vi "SVI_SerialSendAndReceive.vi"(6 "End Char":string="\n", 7 "Wait time (ms)":u32=1000, 8 "error in (no error)":errorcluster, 9 "Tries":i32=50, 10 "Command":string, 11 "VISA Refnum in":refnum<visa-resource-name>) -> (0 "error out":errorcluster, 2 "read buffer":string, 3 "VISA resource name out":refnum<visa-resource-name>)   [LabVIEW 2014]
panel:
  out "Numeric Control":i32
  out "Array":u32[](array[numeric])
  out "Tries":i32
  out "x-y":u32
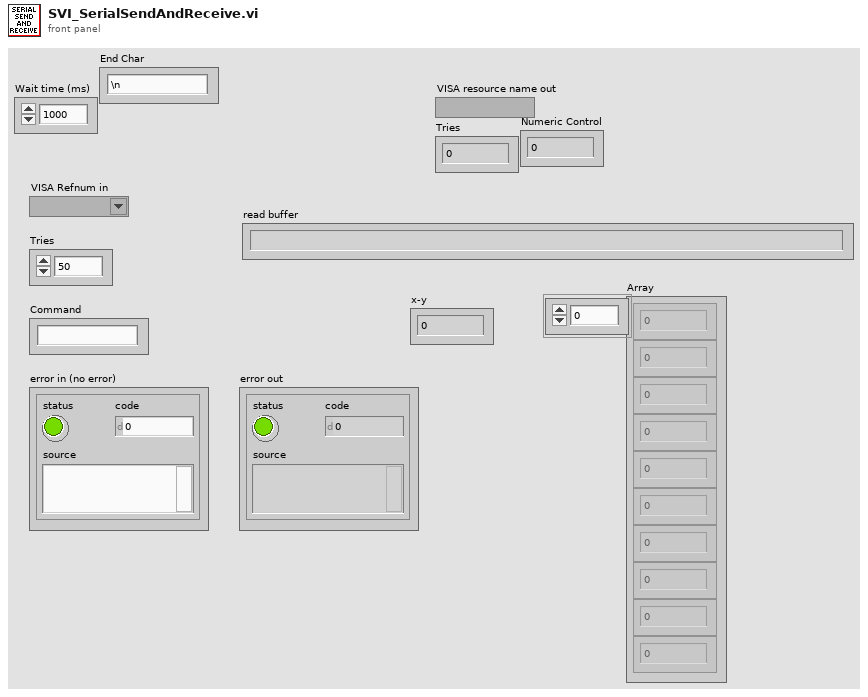
[diagram p1: front panel]
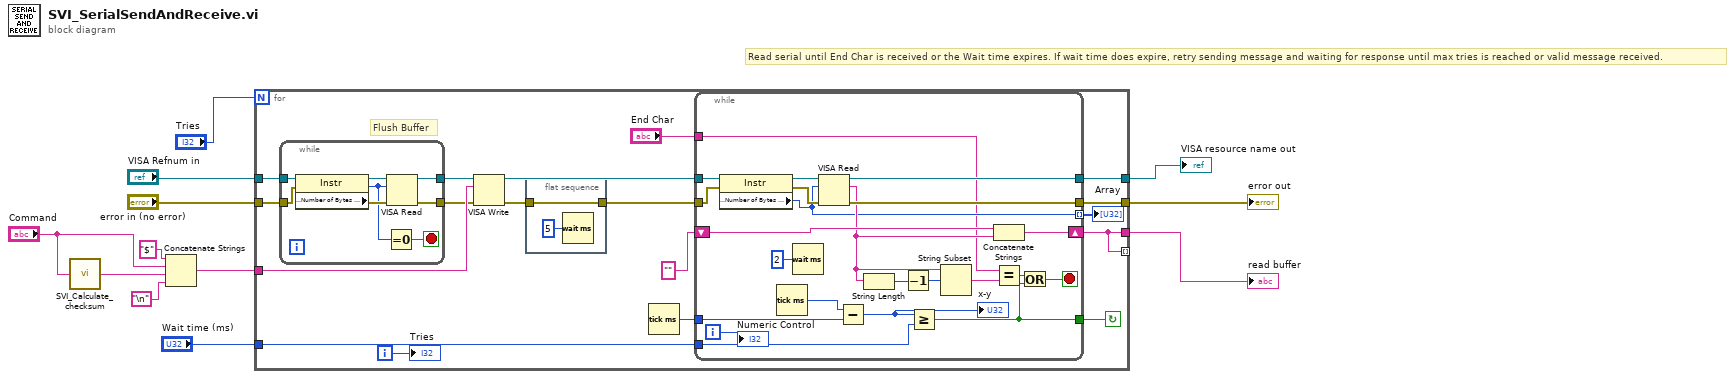
[diagram p0: block diagram]
diagram:
  # "Read serial until End Char is received or the Wait time expires. If wait time does expire, retry sending message and waiting for response until max tries is reached or valid message received."
  n1 = call "SVI_Calculate_checksum.vi"("Message"="Command") -> ("Calculated checksum"=w3:string)
  n2 = Concatenate Strings("$" ("string"), "Command", w3, "\n") -> (w2:string)
  n3 = for {
    N: "Tries" -> [_]
    tunnel: w2 -> [w30]
    tunnel: "VISA Refnum in" -> [w15]
    tunnel: "error in (no error)" -> [w16]
    tunnel: "Wait time (ms)" -> [w26]
    tunnel: [w24] -> w8
    tunnel: [w23] -> w7
    tunnel: [w18] -> w6
    tunnel: [w18] -> _ mode=indexing
    i -> [w22]
    stop <- w25 continue-if-true
    # "Flush Buffer"
    n4 = while {
      tunnel: w15 -> [w34]
      tunnel: [w33] -> w14
      tunnel: w16 -> [w35]
      tunnel: [w36] -> w13
      stop <- w32 stop-if-true
      n5 = property class="Instr"(reference=w34, error in=w35) -> (reference out=w38:refnum<visa-resource-name>, error out=w37:errorcluster, "Serial Settings:Number of Bytes at Serial Port"=w31:u32)
      n6 = Equal To 0?(x=w31) -> (x = 0?=w32:bool)
      n7 = VISA Read(VISA resource name=w38, byte count=w31, error in (no error)=w37) -> (VISA resource name out=w33:refnum<visa-resource-name>, error out=w36:errorcluster)  [unwired: 2 out]
    }
    n8 = VISA Write(VISA resource name=w14, write buffer=w30, error in (no error)=w13) -> (VISA resource name out=w27:refnum<visa-resource-name>, error out=w20:errorcluster)  [unwired: 1 out]
    n9 = flat-sequence {
      tunnel: [w39] -> w19
      tunnel: w20 -> [w39]
      frame #0 {
        n10 = Wait (ms)(milliseconds to wait=u32 5) -> ()  [unwired: 1 out]
      }
    }
    n11 = Tick Count (ms)() -> (millisecond timer value=w29:u32)
    n12 = while {
      tunnel: w27 -> [w61]
      tunnel: [w59] -> w24
      shift-right: [w44] -> w18
      shift-left: "" -> [w57]
      tunnel: w29 -> [w52]
      tunnel: w19 -> [w60]
      tunnel: [w58] -> w23
      tunnel: w26 -> [w48]
      tunnel: [w47] -> w25
      tunnel: [w45] -> w21 mode=indexing
      tunnel: "End Char" -> [w42]
      i -> [w41]
      stop <- w43 stop-if-true
      n13 = property class="Instr"(reference=w61, error in=w60) -> (reference out=w63:refnum<visa-resource-name>, error out=w62:errorcluster, "Serial Settings:Number of Bytes at Serial Port"=w45:u32)
      n14 = Tick Count (ms)() -> (millisecond timer value=w53:u32)
      n15 = Wait (ms)(milliseconds to wait=u32 2) -> ()  [unwired: 1 out]
      n16 = VISA Read(VISA resource name=w63, byte count=w45, error in (no error)=w62) -> (VISA resource name out=w59:refnum<visa-resource-name>, read buffer=w49:string, error out=w58:errorcluster)  [unwired: 1 out]
      n17 = Subtract(x=w53, y=w52) -> (x-y=w51:u32)
      "x-y" <- w51
      n18 = String Length(string=w49) -> (length=w55:i32)
      n19 = Decrement(x=w55) -> (x-1=w54:i32)
      n20 = Greater Or Equal?(x=w51, y=w48) -> (x >= y?=w47:bool)
      n21 = String Subset(string=w49, offset (0)=w54) -> (substring=w50:string)  [unwired: 1 in]
      n22 = Concatenate Strings(w57, w49) -> (w44:string)
      n23 = Equal?(x=w42, y=w50) -> (x = y?=w56:bool)
      n24 = Or(x=w56, y=w47) -> (x .or. y?=w43:bool)
      "Numeric Control" <- w41
    }
    "Array" <- w21
    "Tries" <- w22
  }
  "read buffer" <- w6
  "error out" <- w7
  "VISA resource name out" <- w8
